vi "FindNameInTree.vi"() -> ()   [LabVIEW 2017, in "LVTM.lvlib" / "FindName Task_Manager.lvlib"]
doc: "Provides a mechanism to allow the user to specify a string to be searched for. Tree items containing a match are highlighted. Also, a count of matching tree items is displayed, along with a count of all tree items."
uses:
  FindName Task_Manager.lvlib
  <vilib>/Utility/miscctls.llb/LVSelectionTypeDef.ctl
  LVTM.lvlib
panel:
  in  "Close":bool
  out "Found/Total =":string
  in  "Data Tree":refnum<vi>
  in  "NameToFind":string caption="Find ="
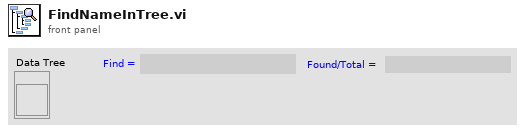
[diagram p1: front panel]
types:
  T1 = typedef "LVSelectionTypeDef.ctl" = cluster{"Selection Start":u32, "Selection End":u32}
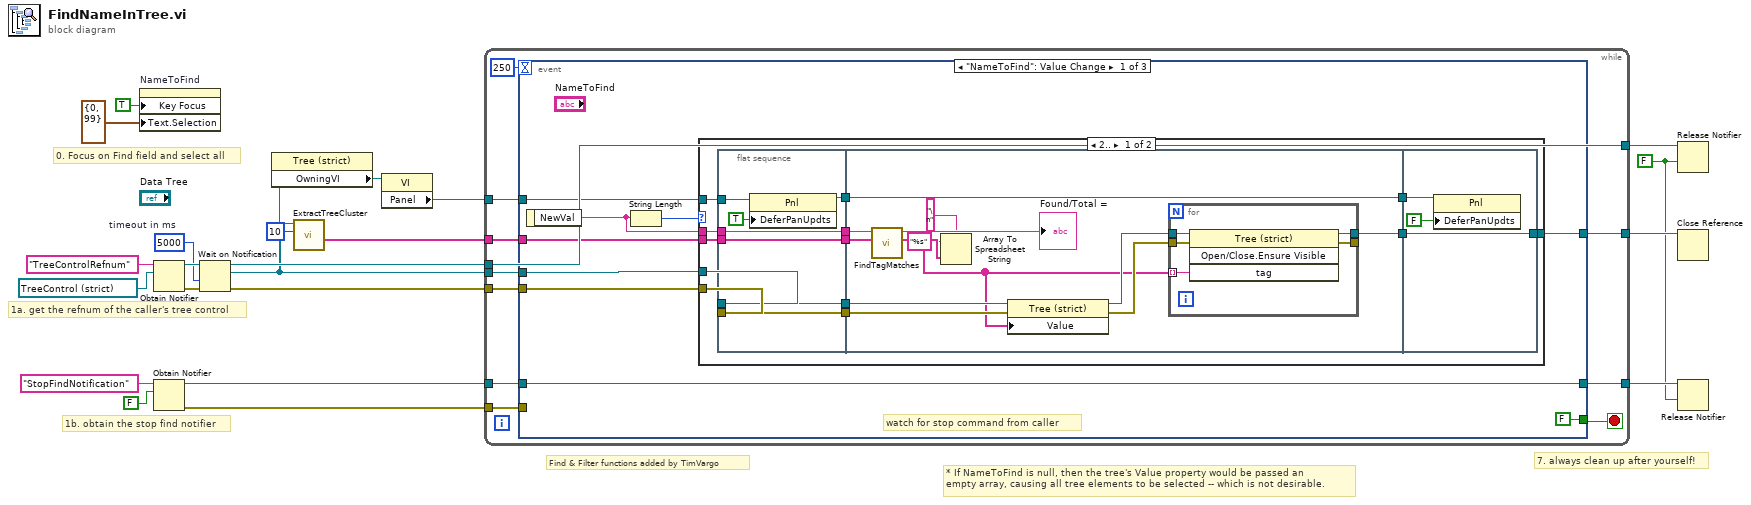
[diagram p0: block diagram]
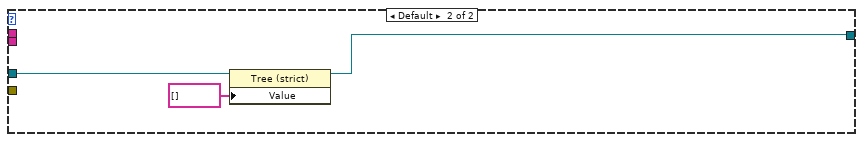
[diagram p2: hidden frame]
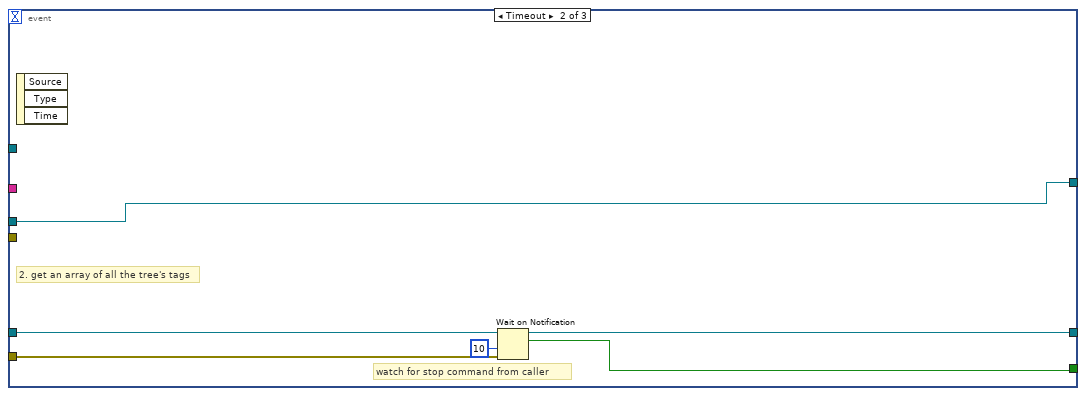
[diagram p3: hidden frame]
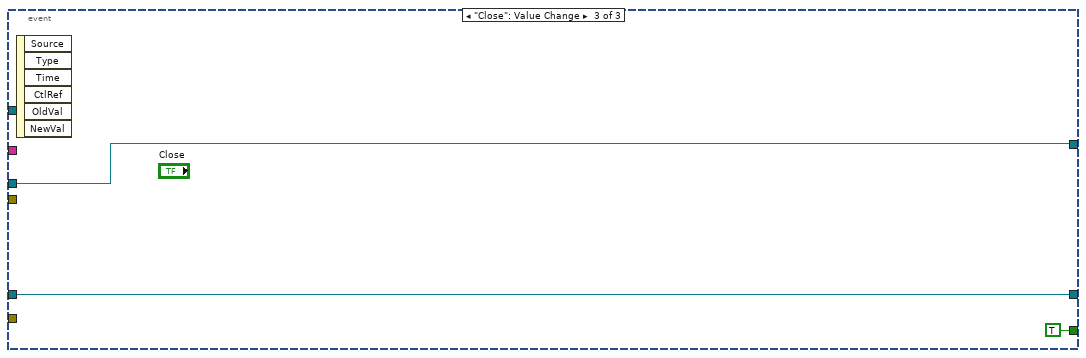
[diagram p4: hidden frame]
diagram:
  w6 = FALSE ("force destroy? (F)")
  w10 = 5000  # timeout in ms
  # "Find & Filter functions added by TimVargo"
  # "* If NameToFind is null, then the tree's Value property would be passed an \nempty array, causing all tree elements to be selected -- which is not desirable."
  # "1b. obtain the stop find notifier"
  # "0. Focus on Find field and select all"
  # "7. always clean up after yourself!"
  # "1a. get the refnum of the caller's tree control"
  n1 = property on="NameToFind" class="Str"("Key Focus"=TRUE, "Text.Selection"=T1 {"Selection Start"=0, "Selection End"=99}) -> ()  [unwired: 2 in, 2 out]
  n2 = Obtain Notifier(name (unnamed)="TreeControlRefnum", notification data type=refnum<vi> refnum ("Data Tree")) -> (notifier out=w19:refnum<notifier>, error out=w20:errorcluster)  [unwired: 2 in, 1 out]
  n3 = Obtain Notifier(name (unnamed)="StopFindNotification", notification data type=FALSE) -> (notifier out=w9:refnum<notifier>, error out=w8:errorcluster)  [unwired: 2 in, 1 out]
  n4 = Wait on Notification(notifier=w19, timeout in ms (-1)=w10, error in (no error)=w20) -> (notifier out=w18:refnum<notifier>, notification=w3:refnum<vi>, error out=w15:errorcluster)  [unwired: 1 in, 1 out]
  n5 = property class="Tree (strict)"(reference=w3) -> ("OwningVI"=w2:refnum<vi>)  [unwired: 1 in, 2 out]
  n6 = call "ExtractTreeCluster.vi"("NumberOfColumns"=10, "TreeReference"=w3) -> ("All Tags"=w4:string[])  [unwired: 6 in, 3 out]
  n7 = property class="VI"(reference=w2) -> ("Panel"=w1:refnum<vi>)  [unwired: 1 in, 2 out]
  n8 = while {
    tunnel: w3 -> [w26]
    tunnel: w18 -> [w33]
    tunnel: [w33] -> w17
    tunnel: [w28] -> w16
    tunnel: w15 -> [w25]
    tunnel: w9 -> [w32]
    tunnel: w8 -> [w31]
    tunnel: [w30] -> w7
    tunnel: w4 -> [w24]
    tunnel: w1 -> [w23]
    stop <- w29 stop-if-true
    n9 = event shown="[0] \"NameToFind\": Value Change" {
      selector: _ -> [_ _ _]
      dyn-events: _ -> [_ _ _]
      timeout: 250 -> [_ _ _]
      tunnel: w26 -> [w41 w86 w92]
      tunnel: w32 -> [w39 w91 w94]
      tunnel: w31 -> [_ w90 _]
      tunnel: [w39 w89 w94] -> w30
      tunnel: [FALSE w87 TRUE] -> w29
      tunnel: [w42 w86 w92] -> w28
      tunnel: w25 -> [w40 _ _]
      tunnel: w24 -> [w37 _ _]
      tunnel: w23 -> [w36 _ _]
      event "NameToFind": Value Change {
        # "watch for stop command from caller"
        n10 = event-data() -> ("NewVal"=w34:string)  [unwired: 1 in]
        n11 = String Length(string=w34) -> (length=w35:i32)
        n12 = case shown="2.." w35 {
          tunnel: [w55 w84] -> w42
          tunnel: w41 -> [w52 w85]
          tunnel: w40 -> [w53 _]
          tunnel: w37 -> [w54 _]
          tunnel: w36 -> [w46 _]
          tunnel: w34 -> [w43 _]
          frame 2.. {
            n13 = flat-sequence {
              tunnel: w52 -> [w59]
              tunnel: w53 -> [w60]
              tunnel: w54 -> [w61]
              tunnel: w43 -> [w62]
              tunnel: [w62] -> w51
              tunnel: [w61] -> w50
              tunnel: [w60] -> w49
              tunnel: [w59] -> w48
              tunnel: w46 -> [w58]
              tunnel: [w57] -> w44
              tunnel: w51 -> [w73]
              tunnel: w50 -> [w69]
              tunnel: w49 -> [w68]
              tunnel: w48 -> [w67]
              tunnel: [w70] -> w47
              tunnel: [w66] -> w45
              tunnel: w44 -> [w66]
              tunnel: [w82] -> w55
              tunnel: w47 -> [w82]
              tunnel: w45 -> [w81]
              frame #0 {
                n14 = property class="Pnl"(reference=w58, "DeferPanUpdts"=TRUE ("Defer Panel Updates")) -> (reference out=w57:refnum<vi>)  [unwired: 1 in, 1 out]
              }
              frame #1 {
                n15 = call "FindTagMatches.vi"("All Tags"=w69, "NameToFind"=w73) -> ("Found"=w65:string[], "ResultString"=→"Found/Total =":string)  [unwired: 7 in, 1 out]
                n16 = Array To Spreadsheet String(delimiter (Tab)="\n", array=w65, 3:"%s" ("format string")) -> ()  [unwired: 1 out]
                n17 = property class="Tree (strict)"(reference=w67, error in=w68, "Value"=w65) -> (reference out=w72:refnum<vi>, error out=w71:errorcluster)
                n18 = for {
                  tunnel: [w79] -> _
                  tunnel: w71 -> [w78]
                  tunnel: w72 -> [w77]
                  tunnel: [w76] -> w70
                  tunnel: w65 -> [w75] mode=indexing
                  n19 = invoke class="Tree (strict)" method="Open/Close.Ensure Visible"(reference=w77, error in=w78, "tag"=w75) -> (reference out=w76:refnum<vi>, error out=w79:errorcluster)  [unwired: 1 in, 2 out]
                }
              }
              frame #2 {
                n20 = property class="Pnl"(reference=w81, "DeferPanUpdts"=FALSE ("Defer Panel Updates")) -> ()  [unwired: 1 in, 2 out]
              }
            }
          }
          frame Default {
            n21 = property class="Tree (strict)"(reference=w85, "Value"=string[] []) -> (reference out=w84:refnum<vi>)  [unwired: 1 in, 1 out]
          }
        }
      }
      event Timeout {
        # "watch for stop command from caller"
        # "2. get an array of all the tree's tags"
        n22 = event-data() -> ()  [unwired: 1 in, 3 out]
        n23 = Wait on Notification(notifier=w91, timeout in ms (-1)=10, error in (no error)=w90) -> (notifier out=w89:refnum<notifier>, notification=w87:bool)  [unwired: 1 in, 2 out]
      }
      event "Close": Value Change {
        n24 = event-data() -> ()  [unwired: 1 in, 6 out]
      }
    }
  }
  n25 = Release Notifier(notifier=w17, force destroy? (F)=w6) -> ()  [unwired: 1 in, 3 out]
  n26 = Close Reference(reference=w16) -> ()  [unwired: 1 in, 1 out]
  n27 = Release Notifier(notifier=w7, force destroy? (F)=w6) -> ()  [unwired: 1 in, 3 out]
